vi "CalcError.vi"(10 "Actual Angle":dbl, 11 "Desired Angle":dbl) -> (2 "ReverseDir?":bool, 3 "Angle Error":dbl)   [LabVIEW 2013, in "ProcessorHelperFunctions.lvlib"]
uses:
  ProcessorHelperFunctions.lvlib
  <vilib>/Analysis/coordinate.llb/Angle Units.ctl
  <vilib>/Analysis/coordinate.llb/Angle Range (Degree).ctl
  <vilib>/Analysis/coordinate.llb/Wrap Angle (scalar).vi
  <vilib>/Analysis/NI_AAL_Angle.lvlib
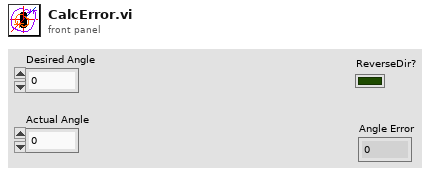
[diagram p1: front panel]
types:
  T1 = typedef "NI_AAL_Angle.lvlib/Angle Range (Degree).ctl" = u16
  T2 = typedef "NI_AAL_Angle.lvlib/Angle Units.ctl" = i32
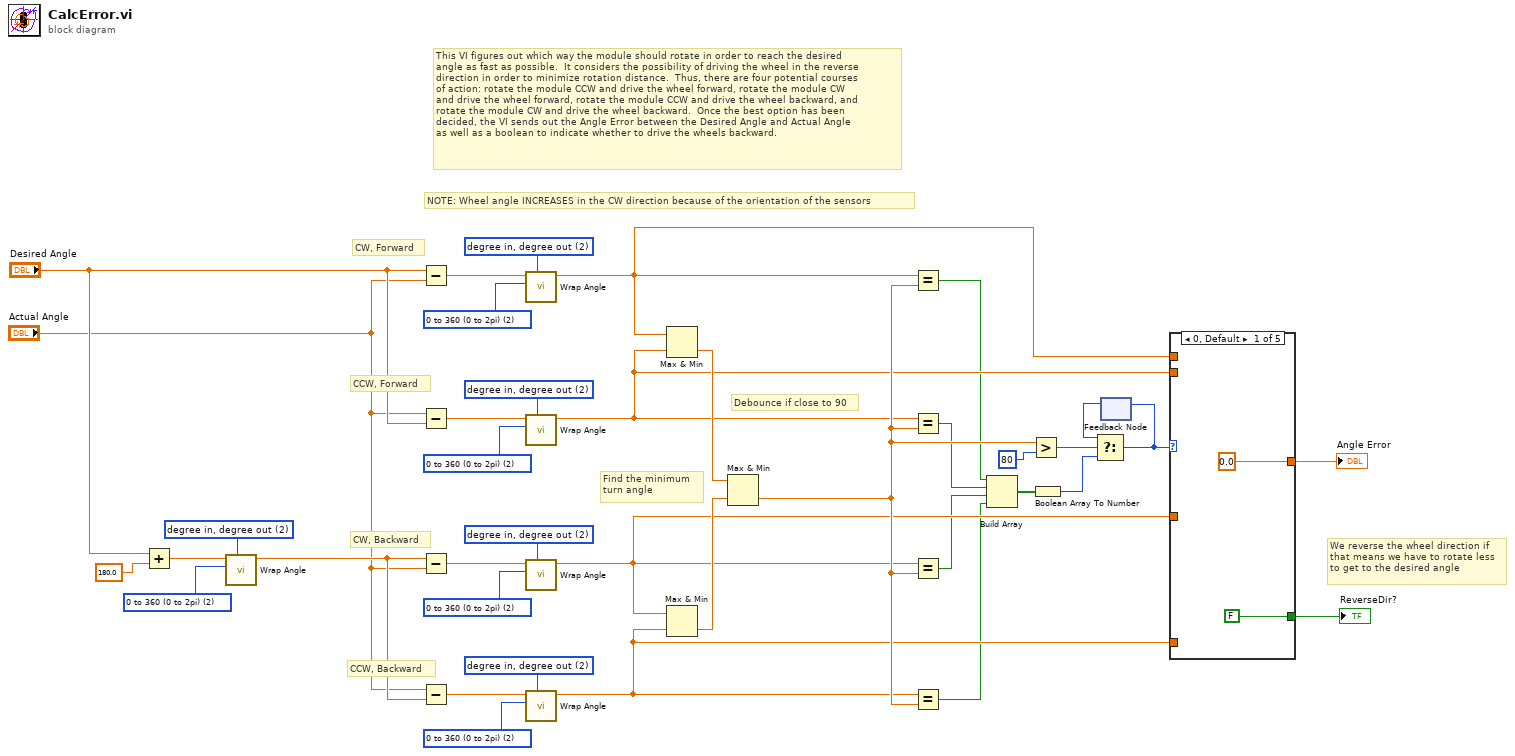
[diagram p0: block diagram]
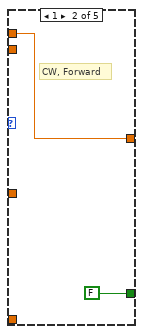
[diagram p2: hidden frame]
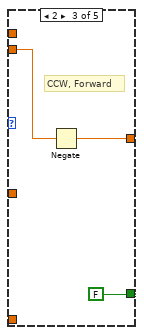
[diagram p3: hidden frame]
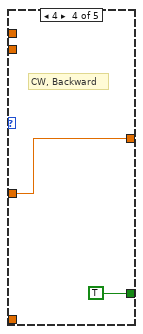
[diagram p4: hidden frame]
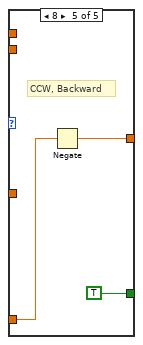
[diagram p5: hidden frame]
diagram:
  w24 = T1 2 items=["none", "-180 to 180 (-pi to pi)", "0 to 360 (0 to 2pi)"] ("angle range")
  w25 = T2 2 items=["radian in, radian out", "radian in, degree out", "degree in, degree out", "degree in, radian out"] ("angle units")
  w26 = T1 2 items=["none", "-180 to 180 (-pi to pi)", "0 to 360 (0 to 2pi)"] ("angle range")
  w27 = T2 2 items=["radian in, radian out", "radian in, degree out", "degree in, degree out", "degree in, radian out"] ("angle units")
  w28 = T1 2 items=["none", "-180 to 180 (-pi to pi)", "0 to 360 (0 to 2pi)"] ("angle range")
  w29 = T2 2 items=["radian in, radian out", "radian in, degree out", "degree in, degree out", "degree in, radian out"] ("angle units")
  w30 = T1 2 items=["none", "-180 to 180 (-pi to pi)", "0 to 360 (0 to 2pi)"] ("angle range")
  w31 = T2 2 items=["radian in, radian out", "radian in, degree out", "degree in, degree out", "degree in, radian out"] ("angle units")
  w36 = T1 2 items=["none", "-180 to 180 (-pi to pi)", "0 to 360 (0 to 2pi)"] ("angle range")
  w37 = T2 2 items=["radian in, radian out", "radian in, degree out", "degree in, degree out", "degree in, radian out"] ("angle units")
  # "NOTE: Wheel angle INCREASES in the CW direction because of the orientation of the sensors"
  # "This VI figures out which way the module should rotate in order to reach the desired\nangle as fast as possible.  It considers the possibility of driving the wheel in the reverse\ndirection in order to minimize rotation distance.  Thus, there are four potential courses\nof action: rotate the module CCW and drive the wheel forward, rotate the module CW\nand drive the wheel forward, rotate the module CCW and drive the wheel backward, and\nrotate the module CW and drive the wheel backward.  Once the best option has been\ndecided, the VI sends out the Angle Error between the Desired Angle and Actual Angle\nas well as a boolean to indicate whether to drive the wheels backward."
  # "We reverse the wheel direction if\nthat means we have to rotate less\nto get to the desired angle"
  # "Find the minimum\nturn angle"
  # "Debounce if close to 90"
  # "CCW, Backward"
  # "CW, Backward"
  # "CCW, Forward"
  # "CW, Forward"
  n1 = Add(x="Desired Angle", y=180.0) -> (x+y=w35:dbl)
  n2 = call-poly <vilib>:"Wrap Angle.vi"("angle units"=w37, "angle range"=w36, "angle in"=w35) -> ("angle out"=w33:dbl)  [unwired: 7 in, 1 out]
  n3 = Subtract(x="Desired Angle", y="Actual Angle") -> (x-y=w19:dbl)
  n4 = Subtract(x="Actual Angle", y="Desired Angle") -> (x-y=w20:dbl)
  n5 = Subtract(x=w33, y="Actual Angle") -> (x-y=w18:dbl)
  n6 = Subtract(x="Actual Angle", y=w33) -> (x-y=w17:dbl)
  n7 = call-poly <vilib>:"Wrap Angle.vi"("angle units"=w31, "angle range"=w30, "angle in"=w19) -> ("angle out"=w11:dbl)  [unwired: 7 in, 1 out]
  n8 = call-poly <vilib>:"Wrap Angle.vi"("angle units"=w29, "angle range"=w28, "angle in"=w20) -> ("angle out"=w12:dbl)  [unwired: 7 in, 1 out]
  n9 = call-poly <vilib>:"Wrap Angle.vi"("angle units"=w27, "angle range"=w26, "angle in"=w18) -> ("angle out"=w10:dbl)  [unwired: 7 in, 1 out]
  n10 = call-poly <vilib>:"Wrap Angle.vi"("angle units"=w25, "angle range"=w24, "angle in"=w17) -> ("angle out"=w9:dbl)  [unwired: 7 in, 1 out]
  n11 = Max & Min(x=w11, y=w12) -> (min(x,y)=w23:dbl)  [unwired: 1 out]
  n12 = Max & Min(x=w10, y=w9) -> (min(x,y)=w22:dbl)  [unwired: 1 out]
  n13 = Max & Min(x=w23, y=w22) -> (min(x,y)=w14:dbl)  [unwired: 1 out]
  n14 = Equal?(x=w11, y=w14) -> (x = y?=w7:bool)
  n15 = Equal?(x=w12, y=w14) -> (x = y?=w8:bool)
  n16 = Equal?(x=w10, y=w14) -> (x = y?=w5:bool)
  n17 = Equal?(x=w9, y=w14) -> (x = y?=w6:bool)
  n18 = Build Array(w7, w8, w5, w6) -> (w21:bool[])
  n19 = Greater?(x=w14, y=80) -> (0:w4:bool)
  n20 = Boolean Array To Number(Boolean array=w21) -> (number=w3:u32)
  n21 = feedback #1() -> (w1:u32)  [unwired: 1 in]
  n22 = Select(t=w1, s=w4, f=w3) -> (s? t:f=w2:u32)
  n23 = feedback-in #1(w2) -> ()
  n24 = case shown="0, Default" w2 {
    tunnel: [FALSE FALSE FALSE TRUE TRUE] -> w16
    tunnel: w12 -> [_ _ w44 _ _]
    tunnel: w11 -> [_ w41 _ _ _]
    tunnel: w10 -> [_ _ _ w46 _]
    tunnel: w9 -> [_ _ _ _ w49]
    tunnel: [0.0 ("angle out") w41 w43 w46 w48] -> w13
    frame 0, Default {
    }
    frame 1 {
      # "CW, Forward"
    }
    frame 2 {
      # "CCW, Forward"
      n25 = Negate(x=w44) -> (-x=w43:dbl)
    }
    frame 4 {
      # "CW, Backward"
    }
    frame 8 {
      # "CCW, Backward"
      n26 = Negate(x=w49) -> (-x=w48:dbl)
    }
  }
  "ReverseDir?" <- w16
  "Angle Error" <- w13
